vi "build_manual_control.vi"(4 "set_manual_control_mode_pedal":bool, 6 "manual_gear":T4, 8 "error in":errorcluster, 11 "Vehicle Control":T1) -> (0 "error out":errorcluster, 3 "manual_control":T2)   [LabVIEW 2019]
doc: "Tool to build a message to control the ego vehicle. Allows to change from autopilot to manual control."
uses:
  controls/Manual Gear.ctl
  controls/Manual Control.ctl
  controls/TorqueControlVehicle.ctl
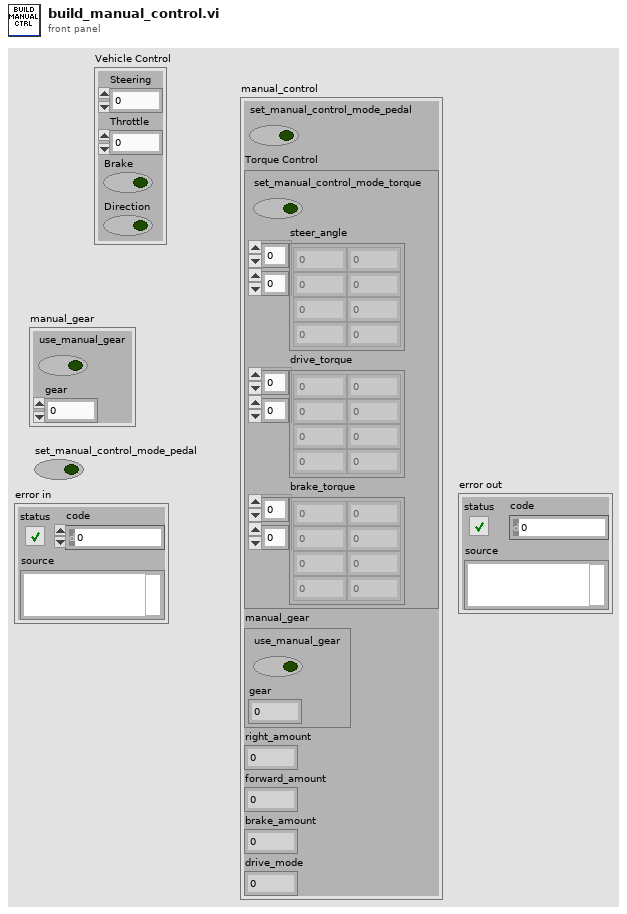
[diagram p1: front panel]
types:
  T1 = cluster{"Steering":sgl, "Throttle":sgl, "Brake":bool, "Direction":bool}
  T2 = typedef "Manual Control.ctl" = cluster{"set_manual_control_mode_pedal":bool, "Torque Control":T3, "manual_gear":T4, "right_amount":sgl, "forward_amount":sgl, "brake_amount":sgl, "drive_mode":i16}
  T3 = typedef "TorqueControlVehicle.ctl" = cluster{"set_manual_control_mode_torque":bool, "steer_angle":sgl[][], "drive_torque":sgl[][], "brake_torque":sgl[][]}
  T4 = typedef "Manual Gear.ctl" = cluster{"use_manual_gear":bool, "gear":i32}
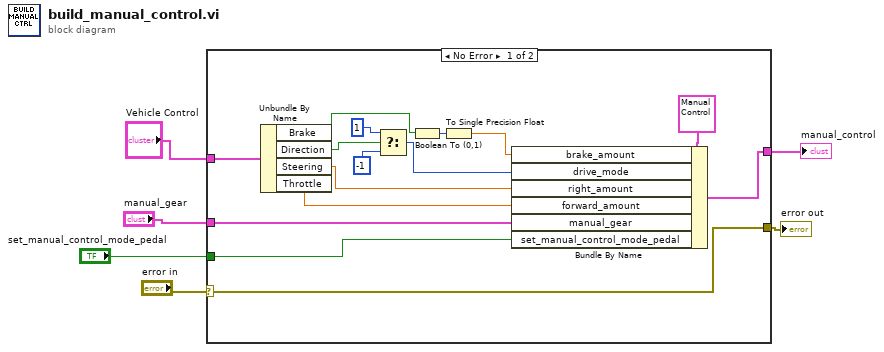
[diagram p0: block diagram]
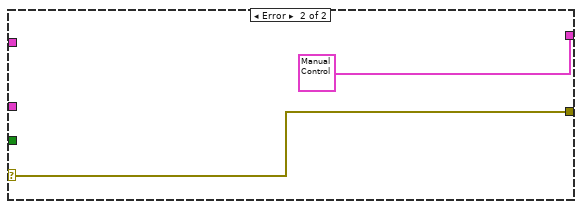
[diagram p2: hidden frame]
diagram:
  n1 = case shown="No Error" "error in" {
    selector: "error in" -> [w21 w23]
    tunnel: [w21 w23] -> w5
    tunnel: [w7 T2 {"set_manual_control_mode_pedal"=TRUE, "Torque Control"={"set_manual_control_mode_torque"=FALSE, "steer_angle"=[[0.0, 0.0], [1.0, 0.0], [2.0, 0.0], [3.0, 0.0]], "drive_torque"=[[0.0, 0.0], [1.0, 0.0], [2.0, 0.0], [3.0, 0.0]], "brake_torque"=[[0.0, 0.0], [1.0, 0.0], [2.0, 0.0], [3.0, 0.0]]}, "manual_gear"={"use_manual_gear"=TRUE, "gear"=2}, "right_amount"=0.0, "forward_amount"=0.0, "brake_amount"=0.0, "drive_mode"=0} ("manual_control")] -> w4
    tunnel: "Vehicle Control" -> [w10 _]
    tunnel: "manual_gear" -> [w9 _]
    tunnel: "set_manual_control_mode_pedal" -> [w8 _]
    frame No Error {
      n2 = Unbundle By Name(w10) -> ("Brake"=w19:bool, "Direction"=w20:bool, "Steering"=w17:sgl, "Throttle"=w18:sgl)
      n3 = Select(t=i16 1, s=w20, f=i16 -1) -> (s? t:f=w15:i16)
      n4 = Boolean To (0,1)(Boolean=w19) -> (0, 1=w14:i16)
      n5 = To Single Precision Float(number=w14) -> (single precision float=w16:sgl)
      n6 = Bundle By Name(cluster=T2 {"set_manual_control_mode_pedal"=TRUE, "Torque Control"={"set_manual_control_mode_torque"=FALSE, "steer_angle"=[[0.0, 0.0], [1.0, 0.0], [2.0, 0.0], [3.0, 0.0]], "drive_torque"=[[0.0, 0.0], [1.0, 0.0], [2.0, 0.0], [3.0, 0.0]], "brake_torque"=[[0.0, 0.0], [1.0, 0.0], [2.0, 0.0], [3.0, 0.0]]}, "manual_gear"={"use_manual_gear"=TRUE, "gear"=2}, "right_amount"=0.0, "forward_amount"=0.0, "brake_amount"=0.0, "drive_mode"=0} ("manual_control"), "brake_amount"=w16, "drive_mode"=w15, "right_amount"=w17, "forward_amount"=w18, "manual_gear"=w9, "set_manual_control_mode_pedal"=w8) -> (w7:T2)
    }
    frame Error {
    }
  }
  "error out" <- w5
  "manual_control" <- w4
